vi "Set Routing Channel States and Connections.vi"(8 "error in (no error)":errorcluster, 10 "Routing Channel States":T1, 11 "Channel Ref in":T4 format="%.0x") -> (0 "error out":errorcluster, 3 "Channel Ref out":T4=18446744073709551615 format="%.0x")   [LabVIEW 2017, in "Switch Scripting.lvlib"]
uses:
  Switch Scripting.lvlib
  <vilib>/NI Veristand/Custom Device API/Custom Device Item Ref.ctl
  Shared/Channel States.ctl
  Shared/Routing State.ctl
  Shared/Connection.ctl
  NationalInstruments.VeriStand.SystemDefinitionAPI
  Utility/Connection to String.vi
  Constants/Scripting Constants.vi
  <vilib>/NI VeriStand/Custom Device API/Custom Device API.lvlib
  Shared/Routing and Faulting Shared.lvlib
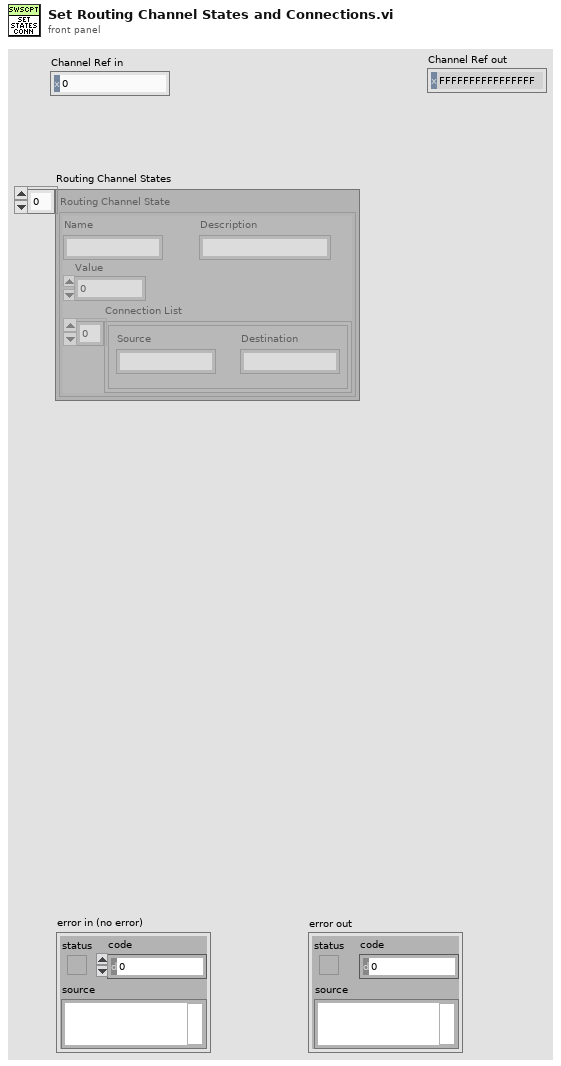
[diagram p1: front panel]
types:
  T1 = typedef "Routing and Faulting Shared.lvlib/Channel States.ctl" = T2[]
  T2 = typedef "Routing and Faulting Shared.lvlib/Routing State.ctl" = cluster{"Name":string, "Description":string, "Value":i32, "Connection List":T3[]}
  T3 = typedef "Routing and Faulting Shared.lvlib/Connection.ctl" = cluster{"Source":string, "Destination":string}
  T4 = typedef "Custom Device API.lvlib/Custom Device Item Ref.ctl" = u64
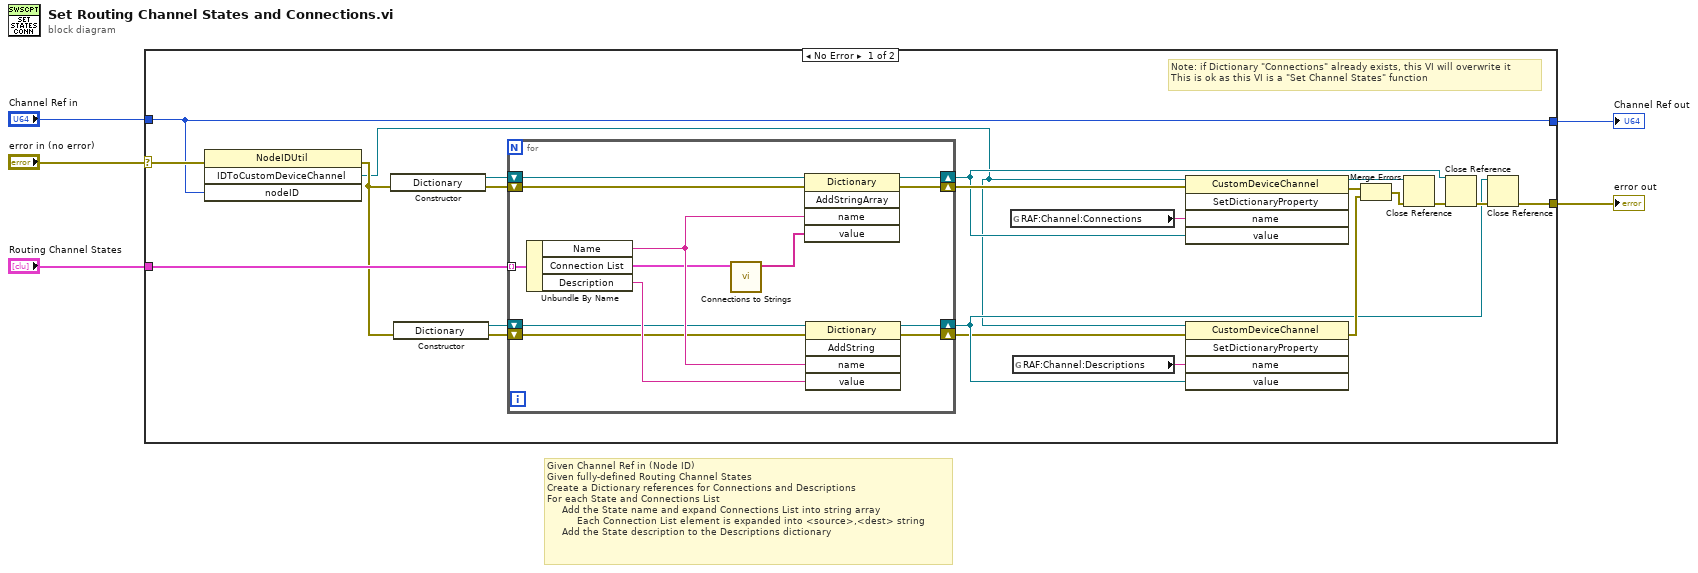
[diagram p0: block diagram]
diagram:
  # "Given Channel Ref in (Node ID)\nGiven fully-defined Routing Channel States\nCreate a Dictionary references for Connections and Descriptions\nFor each State and Connections List\n     Add the State name and expand Connections List into string array\n          Each Connection List element is expanded into <source>,<dest> string\n     Add the State description to the Descriptions dictionary"
  n1 = case shown="No Error" "error in (no error)" {
    selector: "error in (no error)" -> [w27 w42]
    tunnel: [w26 w42] -> w4
    tunnel: "Channel Ref in" -> [w23 w41]
    tunnel: [w23 w41] -> w2
    tunnel: "Routing Channel States" -> [w22 _]
    frame No Error {
      # "Note: if Dictionary \"Connections\" already exists, this VI will overwrite it\nThis is ok as this VI is a \"Set Channel States\" function"
      n2 = invoke class="NodeIDUtil" method="IDToCustomDeviceChannel"(error in=w27, "nodeID"=w23) -> (error out=w7:errorcluster, "IDToCustomDeviceChannel"=w6:refnum<k24>)  [unwired: 2 in, 2 out]
      n3 = constructor class="Dictionary"(error in=w7) -> (reference out=w21:refnum<k24>, error out=w9:errorcluster)  [unwired: 2 in, 1 out]
      n4 = constructor class="Dictionary"(error in=w7) -> (reference out=w20:refnum<k24>, error out=w10:errorcluster)  [unwired: 2 in, 1 out]
      n5 = for {
        tunnel: w22 -> [w40] mode=indexing
        shift-right: [w29] -> w17
        shift-left: w9 -> [w31]
        shift-right: [w37] -> w12
        shift-left: w20 -> [w33]
        shift-right: [w34] -> w13
        shift-left: w21 -> [w32]
        shift-right: [w28] -> w8
        shift-left: w10 -> [w30]
        n6 = Unbundle By Name(w40) -> ("Name"=w39:string, "Connection List"=w36:T3[], "Description"=w38:string)
        n7 = call "Connections to Strings.vi"("connection list"=w36) -> ("connection strings"=w35:string[])  [unwired: 10 in]
        n8 = invoke class="Dictionary" method="AddStringArray"(reference=w32, error in=w31, "name"=w39, "value"=w35) -> (reference out=w34:refnum<k24>, error out=w29:errorcluster)  [unwired: 1 in, 3 out]
        n9 = invoke class="Dictionary" method="AddString"(reference=w33, error in=w30, "name"=w39, "value"=w38) -> (reference out=w37:refnum<k24>, error out=w28:errorcluster)  [unwired: 1 in, 3 out]
      }
      n10 = global read "Scripting Constants.vi" "RAF:Channel:Connections"() -> (w24:string)
      n11 = global read "Scripting Constants.vi" "RAF:Channel:Descriptions"() -> (w11:string)
      n12 = invoke class="CustomDeviceChannel" method="SetDictionaryProperty"(reference=w6, error in=w17, "name"=w24, "value"=w13) -> (reference out=w25:refnum<k24>, error out=w15:errorcluster)  [unwired: 1 in, 3 out]
      n13 = invoke class="CustomDeviceChannel" method="SetDictionaryProperty"(reference=w6, error in=w8, "name"=w11, "value"=w12) -> (error out=w16:errorcluster)  [unwired: 1 in, 4 out]
      n14 = Merge Errors(w15, w16) -> (w14:errorcluster)
      n15 = Close Reference(reference=w25, error in (no error)=w14) -> (error out=w19:errorcluster)
      n16 = Close Reference(reference=w13, error in (no error)=w19) -> (error out=w18:errorcluster)
      n17 = Close Reference(reference=w12, error in (no error)=w18) -> (error out=w26:errorcluster)
    }
    frame Error {
    }
  }
  "Channel Ref out" <- w2
  "error out" <- w4
